vi "Posicion_limite_auto.vi"() -> ()   [LabVIEW 2020]
panel:
  out "Limites posicion auto":T1
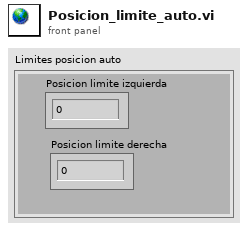
[diagram p1: front panel]
types:
  T1 = cluster{"Posicion limite izquierda":i32, "Posicion limite derecha":i32}
diagram:
